vi "Define User String.vi"(7 "String Value":string, 8 "error in (no error)":errorcluster, 9 "String Name":string, 10 "Operation (0: Add)":i32(ring) items=["Add", "Delete"], 11 "VISA resource name":refnum<visa-resource-name>) -> (0 "error out":errorcluster, 3 "VISA resource name out":refnum<visa-resource-name>)   [LabVIEW 2019, in "Keithley 2600 Series.lvlib"]
doc: "Creates or deletes a user-defined string in nonvolatile memory."
uses:
  Keithley 2600 Series.lvlib
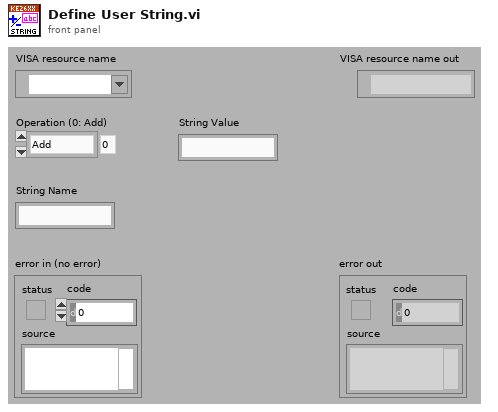
[diagram p1: front panel]
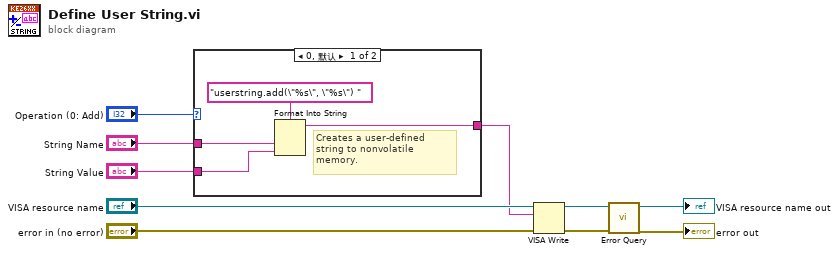
[diagram p0: block diagram]
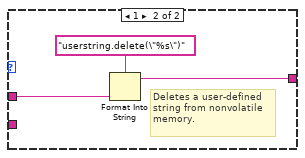
[diagram p2: hidden frame]
diagram:
  n1 = case shown="0, 默认" "Operation (0: Add)" {
    tunnel: "String Name" -> [w13 w16]
    tunnel: "String Value" -> [w12 _]
    tunnel: [w11 w15] -> w1
    frame 0, Default {
      # "Creates a user-defined string to nonvolatile memory."
      n2 = Format Into String(format string="userstring.add(\"%s\", \"%s\") ", w13, w12) -> (resulting string=w11:string)  [unwired: 2 in, 1 out]
    }
    frame 1 {
      # "Deletes a user-defined string from nonvolatile memory."
      n3 = Format Into String(format string="userstring.delete(\"%s\")", w16) -> (resulting string=w15:string)  [unwired: 2 in, 1 out]
    }
  }
  n4 = VISA Write(VISA resource name="VISA resource name", write buffer=w1, error in (no error)="error in (no error)") -> (VISA resource name out=w8:refnum<visa-resource-name>, error out=w7:errorcluster)  [unwired: 1 out]
  n5 = call "Error Query.vi"("error in (no error)"=w7, "VISA resource name"=w8) -> ("error out"=→"error out":errorcluster, "VISA resource name out"=→"VISA resource name out":refnum<visa-resource-name>)  [unwired: 6 in, 2 out]
